vi "Remove_TrainedData.vi"(10 "File Path Control":path, 11 "TrainnedData":string) -> ()   [LabVIEW 2019]
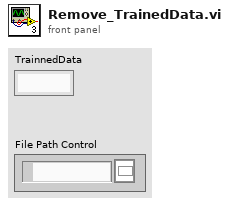
[diagram p1: front panel]
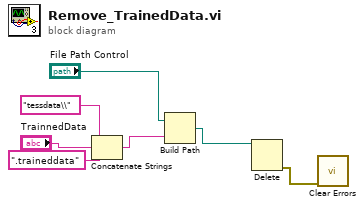
[diagram p0: block diagram]
diagram:
  n1 = Concatenate Strings("tessdata\\" ("string"), "TrainnedData", ".traineddata" ("string")) -> (w2:string)
  n2 = Build Path(base path="File Path Control", name or relative path=w2) -> (appended path=w6:path)
  n3 = Delete(path (use dialog)=w6) -> (error out=w5:errorcluster)  [unwired: 4 in, 2 out]
  n4 = call <vilib>:"Clear Errors.vi"("error in (no error)"=w5) -> ()  [unwired: 5 in, 2 out]
